vi "LCR_InsertMeasurements.vi"(4 "Data Cluster":T3, 6 "TimeStamp":timestamp, 8 "error in (no error)":errorcluster, 9 "Data_IN":T4 {"GUI Data Cluster"."SBR" format="%08b"}, 10 "Cluster IN":T1={"General"={"Config.ini"=path "", "Default Logging Path"=path ""}, "Hardware"={"AHC VISA COM"="", "Measure Rate (1/s)"=0, "Global T VAR"="", "Global B VAR"=""}, "Operation"={"Operation Mode"=enum."Idle-Off", "Status"="", "NewLog?"=FALSE}}) -> (0 "error out":errorcluster, 1 "Data_OUT":T4 {"GUI Data Cluster"."SBR" format="%08b"}, 2 "Cluster OUT":T1={"General"={"Config.ini"=path "", "Default Logging Path"=path ""}, "Hardware"={"AHC VISA COM"="", "Measure Rate (1/s)"=0, "Global T VAR"="", "Global B VAR"=""}, "Operation"={"Operation Mode"=enum."Idle-Off", "Status"="", "NewLog?"=FALSE}})   [LabVIEW 2021]
uses:
  Measurement_Cluster.ctl
  Data_Cluster.ctl
  Mode_Enum.ctl
  Config_Cluster.ctl
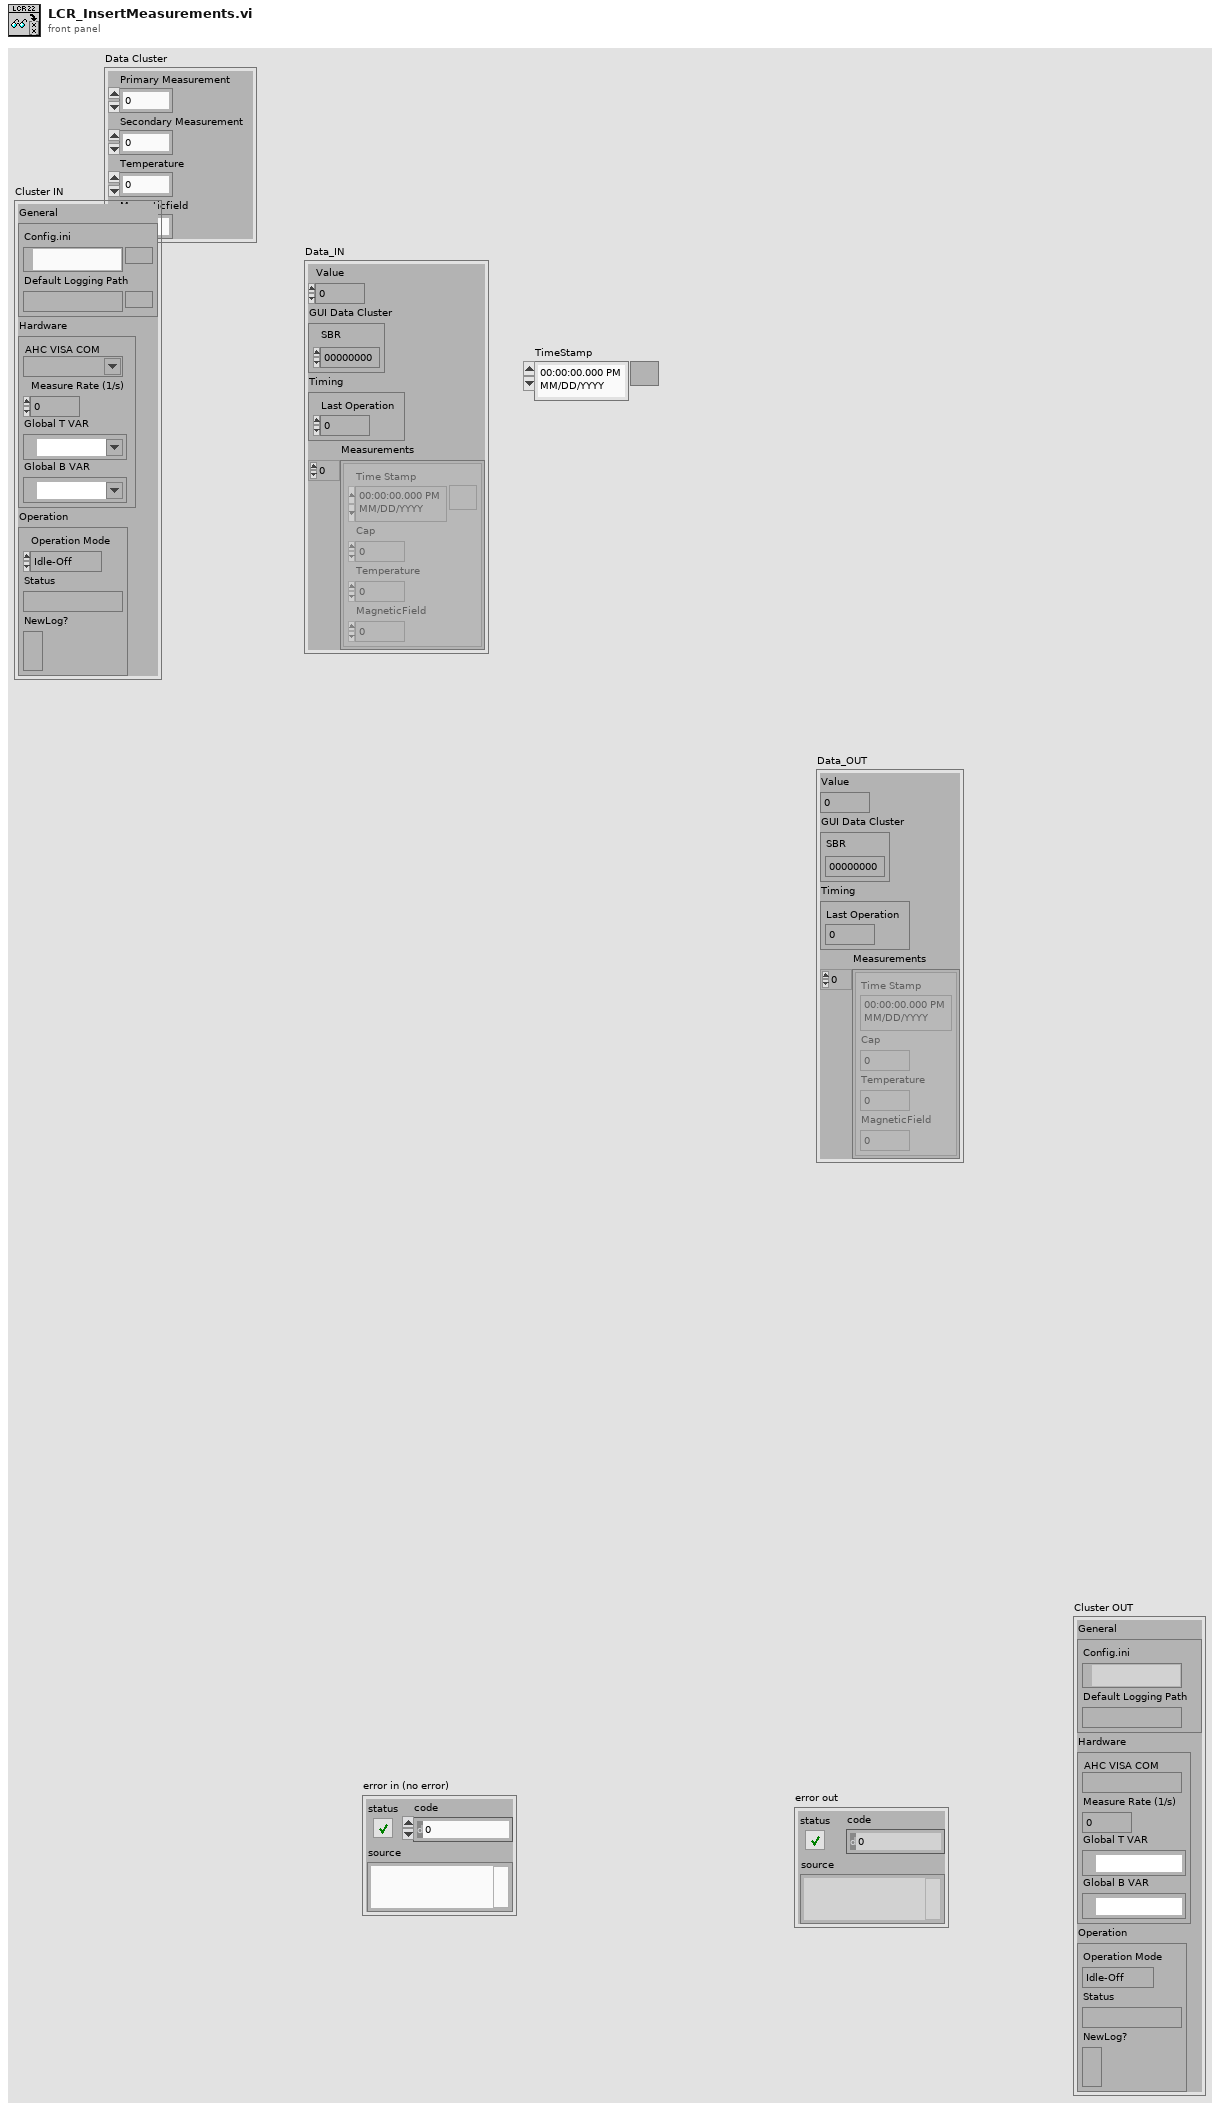
[diagram p1: front panel]
types:
  T1 = typedef "Config_Cluster.ctl" = cluster{"General":cluster{"Config.ini":path, "Default Logging Path":path}, "Hardware":cluster{"AHC VISA COM":refnum<visa-resource-name>, "Measure Rate (1/s)":i32, "Global T VAR":refnum<k21>, "Global B VAR":refnum<k21>}, "Operation":cluster{"Operation Mode":T2, "Status":string, "NewLog?":bool}}
  T2 = typedef "Mode_Enum.ctl" = enum16{"Logging", "Idle-Off", "Idle"}
  T3 = cluster{"Primary Measurement":dbl, "Secondary Measurement":dbl, "Temperature":dbl, "Magneticfield":dbl}
  T4 = typedef "Data_Cluster.ctl" = cluster{"Value":dbl, "GUI Data Cluster":cluster{"SBR":u16}, "Timing":cluster{"Last Operation":dbl}, "Measurements":T5[]}
  T5 = typedef "Measurement_Cluster.ctl" = cluster{"Time Stamp":timestamp, "Cap":dbl, "Temperature":dbl, "MagneticField":dbl}
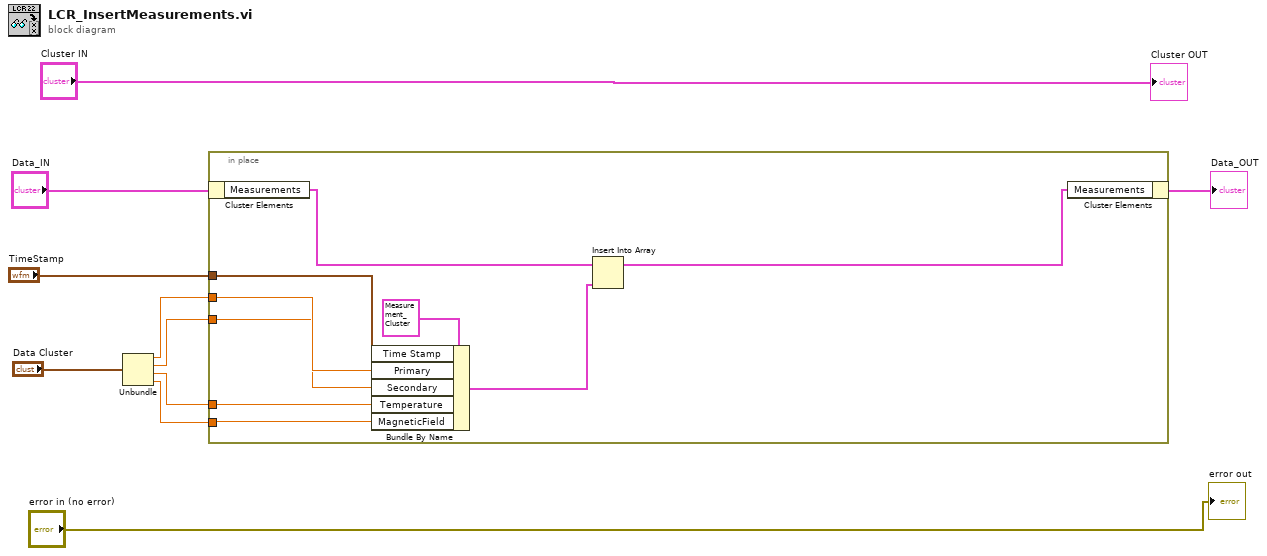
[diagram p0: block diagram]
diagram:
  n1 = Unbundle("Data Cluster") -> ("Primary Measurement"=w6:dbl, "Secondary Measurement"=w5:dbl, "Temperature"=w4:dbl, "Magneticfield"=w3:dbl)
  n2 = in-place {
    in-place-border: "TimeStamp" -> [w17]
    in-place-border: w6 -> [w16]
    in-place-border: w5 -> [w15]
    in-place-border: w4 -> [w12]
    in-place-border: w3 -> [w11]
    n3 = in-place-cluster #1("Data_IN") -> ("Measurements"=w19:T5[])
    n4 = Bundle By Name(cluster=T5 {"Time Stamp"=timestamp(0 s since 1904-01-01), "Cap"=0.0, "Temperature"=0.0, "MagneticField"=0.0} ("new element/subarray"), "Time Stamp"=w17, "Primary"=w16, "Secondary"=w15, "Temperature"=w12, "MagneticField"=w11) -> (w14:T5)
    n5 = Insert Into Array(array=w19, new element=w14) -> (w13:T5[])  [unwired: 1 in]
    n6 = in-place-cluster #1("Measurements"=w13) -> (→"Data_OUT":T4)
  }
  "Cluster OUT" <- "Cluster IN"
  "error out" <- "error in (no error)"
